vi "Main.Cleanup.vi"(11 "State Variables":T1={"Main"={"FPGA.Session"=0, "Incoming.Decimation"=0, "Outgoing.Decimation"=0, "Process"=refnum}, "Protocol"={"Name"="", "XNET.Settings"={"Database"="", "Cluster"="", "Port"="", "Baud rate [Bd]"=0, "Termination"=0, "Incoming Decimation"=0, "Outgoing Decimation"=1}, "Monitor.Network"={"Address"=0, "Name"=0, "Include DA"=FALSE, "Force SA"=FALSE}, "Data"=[], "DTCs"=[], "Sim.Nodes.LUT"=variant, "Data.LUT"=variant, "PCL"=0}} {"Protocol"."Monitor.Network"."Name" format="%.0x"; "Protocol"."Data"."Trigger.Refs"."Data Reference" format="%.0x"; "Protocol"."Data"."Disable.Refs"."Data Reference" format="%.0x"; "Protocol"."Data"."Timing.Refs"."Data Reference" format="%.0x"; "Protocol"."Data"."Network"."Name" format="%.0x"; "Protocol"."Data"."Incoming.Refs"."Data Reference" format="%.0x"; "Protocol"."Data"."Outgoing.Refs"."Data Reference" format="%.0x"; "Protocol"."XNET.Settings"."Termination" items=["Off", "On"]}) -> (0 "error out":errorcluster)   [LabVIEW 2023, in "J1939 Addon Engine.lvlib"]
uses:
  J1939 Addon Engine.lvlib
  Types/Main.State Variables.ctl
  <vilib>/NI/NIVS Inline Async API/_VS Inline Async API/VS Inline Async API/VS Inline Async API.lvclass
  Types/Main.Settings.ctl
  Types/Protocol.App Settings.ctl
  Addon Shared/Types/XNET Settings.ctl
  Addon Shared/Types/Monitor Settings.ctl
  Types/Protocol.XNET Refs.ctl
  <vilib>/NI VeriStand/Custom Device API/Block Data Reference.ctl
  <vilib>/NI VeriStand/Custom Device API/Data Reference.ctl
  Types/Main.Outgoing.Frame.Settings.ctl
  Addon Shared/Types/Outgoing Event Trigger Types.ctl
  SubModules/Frame-Protection-Support/Source/Shared/Types/Exported Frame Settings.ctl
  SubModules/Frame-Protection-Support/Source/Shared/Types/Exported Frame Type.ctl
  SubModules/Frame-Protection-Support/Source/Shared/Types/Exported Protection Settings.ctl
  SubModules/Frame-Protection-Support/Source/Shared/Types/Protection Type.ctl
  SubModules/Frame-Protection-Support/Source/Shared/Types/XNET Signal Configuration.ctl
  SubModules/Frame-Protection-Support/Source/Shared/Types/Exported Counter Settings.ctl
  SubModules/Frame-Protection-Support/Source/Shared/Types/Exported Event Trigger Type.ctl
  Types/Engine.DTC Settings.ctl
  Addon Shared/Types/Compiled Simulated Settings.ctl
  Types/Engine.DTC FIFOs.ctl
  <vilib>/xnet/xnet.llb/XNET Database Close (Database).vi
  <vilib>/NI VeriStand/Custom Device API/Custom Device API.lvlib
  Addon Shared/J1939 Addon Shared.lvlib
  SubModules/Frame-Protection-Support/Source/Shared/Protection and Counter Support Shared.lvlib
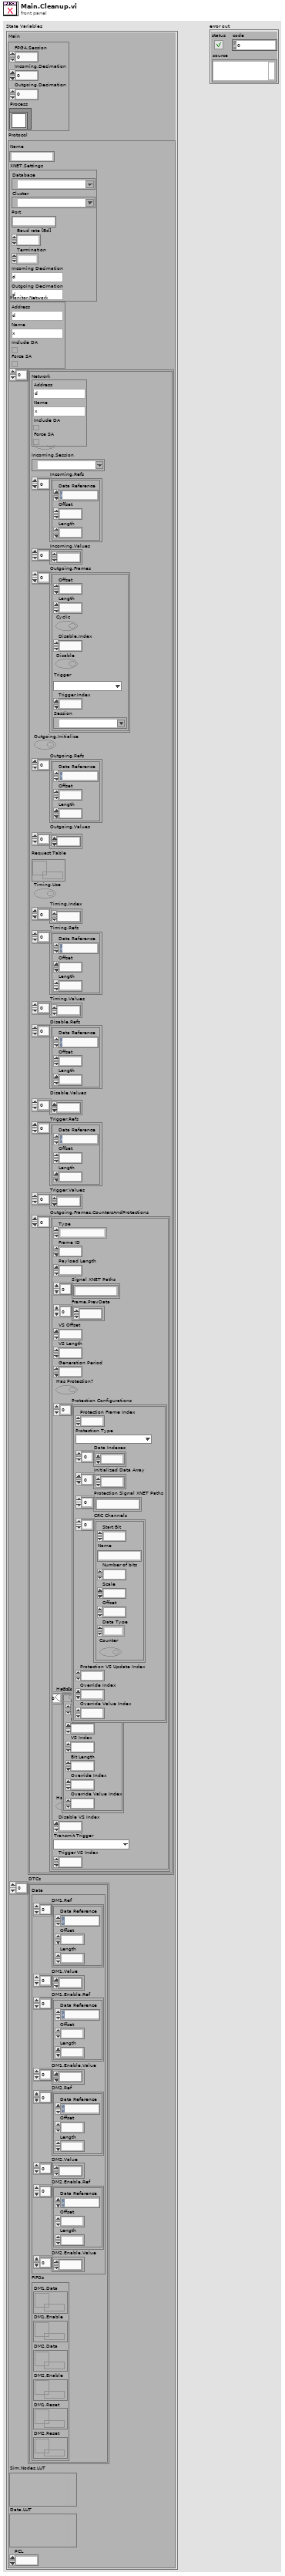
[diagram p1: front panel]
types:
  T1 = typedef "J1939 Addon Engine.lvlib/Main.State Variables.ctl" = cluster{"Main":T2, "Protocol":T3}
  T2 = typedef "J1939 Addon Engine.lvlib/Main.Settings.ctl" = cluster{"FPGA.Session":u32, "Incoming.Decimation":u32, "Outgoing.Decimation":u32, "Process":refnum<class "VS Inline Async API.lvclass">}
  T3 = typedef "J1939 Addon Engine.lvlib/Protocol.App Settings.ctl" = cluster{"Name":string, "XNET.Settings":T4, "Monitor.Network":T5, "Data":T6[], "DTCs":T18[], "Sim.Nodes.LUT":variant, "Data.LUT":variant, "PCL":u32}
  T4 = typedef "J1939 Addon Shared.lvlib/XNET Settings.ctl" = cluster{"Database":refnum<k21>, "Cluster":refnum<k21>, "Port":string, "Baud rate [Bd]":u32, "Termination":u32, "Incoming Decimation":u32, "Outgoing Decimation":u32}
  T5 = typedef "J1939 Addon Shared.lvlib/Monitor Settings.ctl" = cluster{"Address":u8, "Name":u64, "Include DA":bool, "Force SA":bool}
  T6 = typedef "J1939 Addon Engine.lvlib/Protocol.XNET Refs.ctl" = cluster{"Network":T5, "Incoming.Use":bool, "Incoming.Session":refnum<k21>, "Incoming.Refs":T7[], "Incoming.Values":dbl[], "Outgoing.Frames":T9[], "Outgoing.Initialize":bool, "Outgoing.Refs":T7[], "Outgoing.Values":dbl[], "Request.Table":refnum<k33>, "Timing.Use":bool, "Timing.Index":i32[], "Timing.Refs":T7[], "Timing.Values":dbl[], "Disable.Refs":T7[], "Disable.Values":dbl[], "Trigger.Refs":T7[], "Trigger.Values":dbl[], "Outgoing.Frames.CountersAndProtections":T11[]}
  T7 = typedef "Custom Device API.lvlib/Block Data Reference.ctl" = cluster{"Data Reference":T8, "Offset":u64, "Length":u64}
  T8 = typedef "Custom Device API.lvlib/Data Reference.ctl" = i32
  T9 = typedef "J1939 Addon Engine.lvlib/Main.Outgoing.Frame.Settings.ctl" = cluster{"Offset":u32, "Length":u32, "Cyclic":bool, "Disable.Index":i32, "Disable":bool, "Trigger":T10, "Trigger.Index":i32, "Session":refnum<k21>}
  T10 = typedef "J1939 Addon Shared.lvlib/Outgoing Event Trigger Types.ctl" = enum16{"Channel value change", "Trigger channel (not zero)", "Channel value change or trigger channel (not zero)", "Trigger channel (any value change)", "Channel value change or trigger channel (any value change)"}
  T11 = typedef "Protection and Counter Support Shared.lvlib/Exported Frame Settings.ctl" = cluster{"Type":T12, "Frame ID":u32, "Payload Length":u32, "Signal XNET Paths":string[], "Frame.PrevData":dbl[], "VS Offset":i32, "VS Length":i32, "Generation Period":u32, "Has Protection?":bool, "Protection Configurations":T13[], "Has Counter":bool, "Counter Configurations":T16[], "Has Disable?":bool, "Disable VS Index":i32, "Transmit Trigger":T17, "Trigger VS Index":i32}
  T12 = typedef "Protection and Counter Support Shared.lvlib/Exported Frame Type.ctl" = enum16{"Periodic", "Event", "Periodic/Event"}
  T13 = typedef "Protection and Counter Support Shared.lvlib/Exported Protection Settings.ctl" = cluster{"Protection Frame Index":i32, "Protection Type":T14, "Data Indeces":i32[], "Initialized Data Array":dbl[], "Protection Signal XNET Paths":string[], "CRC Channels":T15[], "Protection VS Update Index":i32, "Override Index":i32, "Override Value Index":i32}
  T14 = typedef "Protection and Counter Support Shared.lvlib/Protection Type.ctl" = enum16{"Arb ID + Bytes Checksum with Inversion", "Arb ID + Bytes CRC with Inversion", "Reversed Raw Signal Checksum with Inversion", "Concatenated Two's Compliment"}
  T15 = typedef "Protection and Counter Support Shared.lvlib/XNET Signal Configuration.ctl" = cluster{"Start Bit":i32, "Name":string, "Number of bits":i32, "Scale":dbl, "Offset":dbl, "Data Type":u32, "Counter":bool}
  T16 = typedef "Protection and Counter Support Shared.lvlib/Exported Counter Settings.ctl" = cluster{"Frame Index":i32, "Max Count":dbl, "VS Index":i32, "Bit Length":i64, "Override Index":i32, "Override Value Index":i32}
  T17 = typedef "Protection and Counter Support Shared.lvlib/Exported Event Trigger Type.ctl" = enum16{"Channel value change", "Trigger channel (not zero)", "Channel value change or trigger channel (not zero)", "Trigger channel (any value change)", "Channel value change or trigger channel (any value change)"}
  T18 = typedef "J1939 Addon Engine.lvlib/Engine.DTC Settings.ctl" = cluster{"Data":T19, "FIFOs":T20}
  T19 = typedef "J1939 Addon Shared.lvlib/Compiled Simulated Settings.ctl" = cluster{"DM1.Ref":T7[], "DM1.Value":dbl[], "DM1.Enable.Ref":T7[], "DM1.Enable.Value":dbl[], "DM2.Ref":T7[], "DM2.Value":dbl[], "DM2.Enable.Ref":T7[], "DM2.Enable.Value":dbl[]}
  T20 = typedef "J1939 Addon Engine.lvlib/Engine.DTC FIFOs.ctl" = cluster{"DM1.Data":refnum<k33>, "DM1.Enable":refnum<k33>, "DM2.Data":refnum<k33>, "DM2.Enable":refnum<k33>, "DM1.Reset":refnum<k33>, "DM2.Reset":refnum<k33>}
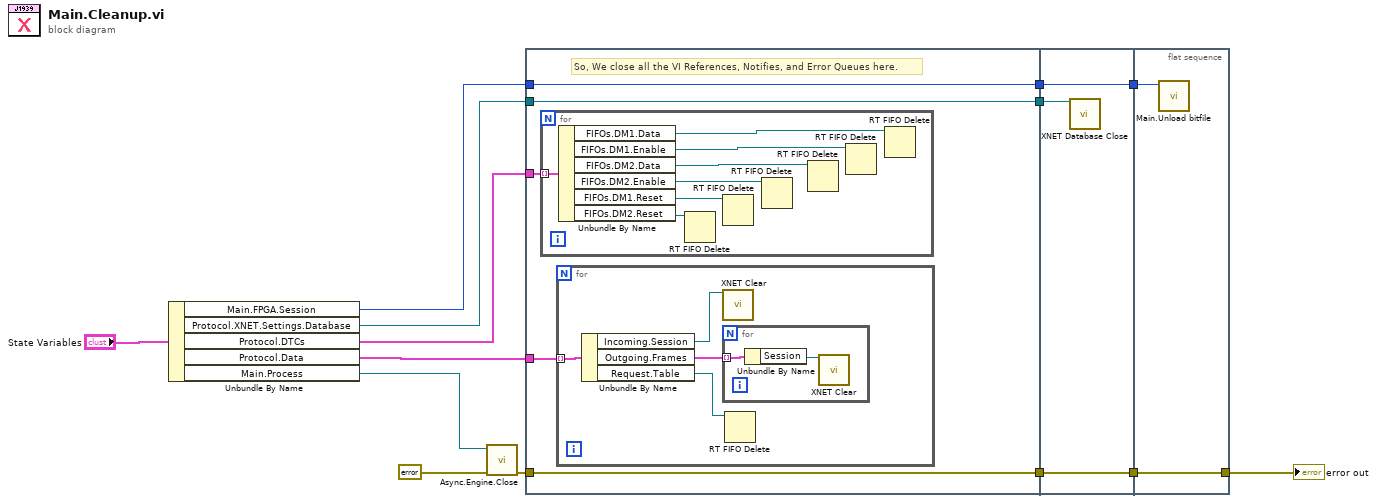
[diagram p0: block diagram]
diagram:
  n1 = Unbundle By Name("State Variables") -> ("Main.FPGA.Session"=w5:u32, "Protocol.XNET.Settings.Database"=w8:refnum<k21>, "Protocol.DTCs"=w9:T18[], "Protocol.Data"=w6:T6[], "Main.Process"=w3:refnum<class "VS Inline Async API.lvclass">)
  n2 = call <vilib>:"Async.Engine.Close.vi"("error in (no error)"=errorcluster {"status"=FALSE, "code"=0, "source"=""}, "Async in"=w3) -> ("error out"=w4:errorcluster)  [unwired: 8 in, 1 out]
  n3 = flat-sequence {
    tunnel: w4 -> [w19]
    tunnel: w8 -> [w18]
    tunnel: [w19] -> w14
    tunnel: [w18] -> w13
    tunnel: [w17] -> w12
    tunnel: w5 -> [w17]
    tunnel: w9 -> [w16]
    tunnel: w6 -> [w15]
    tunnel: w14 -> [w35]
    tunnel: w13 -> [w34]
    tunnel: [w35] -> w11
    tunnel: [w33] -> w10
    tunnel: w12 -> [w33]
    tunnel: [w37] -> w2
    tunnel: w11 -> [w37]
    tunnel: w10 -> [w36]
    frame #0 {
      # "So, We close all the VI References, Notifies, and Error Queues here."
      n4 = for {
        tunnel: w16 -> [w26] mode=indexing
        n5 = Unbundle By Name(w26) -> ("FIFOs.DM1.Data"=w25:refnum<k33>, "FIFOs.DM1.Enable"=w24:refnum<k33>, "FIFOs.DM2.Data"=w23:refnum<k33>, "FIFOs.DM2.Enable"=w20:refnum<k33>, "FIFOs.DM1.Reset"=w21:refnum<k33>, "FIFOs.DM2.Reset"=w22:refnum<k33>)
        n6 = RT FIFO Delete(0:w22) -> ()  [unwired: 2 in, 1 out]
        n7 = RT FIFO Delete(0:w21) -> ()  [unwired: 2 in, 1 out]
        n8 = RT FIFO Delete(0:w20) -> ()  [unwired: 2 in, 1 out]
        n9 = RT FIFO Delete(0:w23) -> ()  [unwired: 2 in, 1 out]
        n10 = RT FIFO Delete(0:w24) -> ()  [unwired: 2 in, 1 out]
        n11 = RT FIFO Delete(0:w25) -> ()  [unwired: 2 in, 1 out]
      }
      n12 = for {
        tunnel: w15 -> [w28] mode=indexing
        n13 = Unbundle By Name(w28) -> ("Incoming.Session"=w30:refnum<k21>, "Outgoing.Frames"=w29:T9[], "Request.Table"=w27:refnum<k33>)
        n14 = call <vilib>:"XNET Clear.vi"("session in"=w30) -> ()  [unwired: 14 in, 1 out]
        n15 = for {
          tunnel: w29 -> [w32] mode=indexing
          n16 = Unbundle By Name(w32) -> ("Session"=w31:refnum<k21>)
          n17 = call <vilib>:"XNET Clear.vi"("session in"=w31) -> ()  [unwired: 14 in, 1 out]
        }
        n18 = RT FIFO Delete(0:w27) -> ()  [unwired: 2 in, 1 out]
      }
    }
    frame #1 {
      n19 = call-poly <vilib>:"XNET Database Close.vi"("database in"=w34) -> ()  [unwired: 14 in, 1 out]
    }
    frame #2 {
      n20 = call "Main.Unload bitfile.vi"("Session"=w36) -> ()  [unwired: 11 in]
    }
  }
  "error out" <- w2
